vi "median filter.vi"(10 "Sample Length":i32=5, 11 "Element Input":dbl) -> (3 "Output Element":dbl)   [LabVIEW 2016]
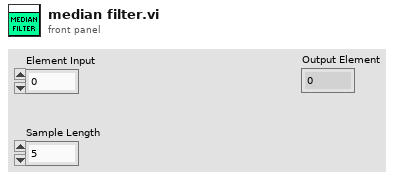
[diagram p1: front panel]
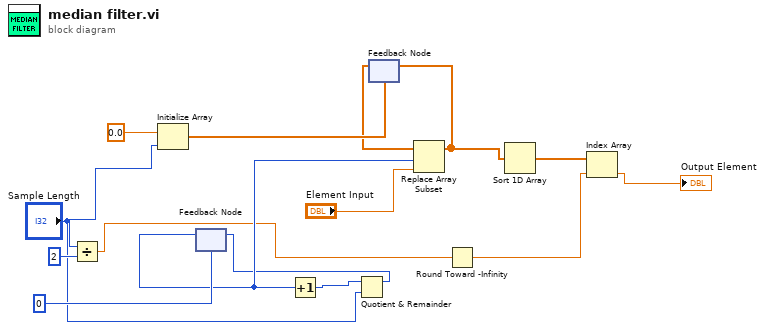
[diagram p0: block diagram]
diagram:
  n1 = Divide(x="Sample Length", y=2) -> (x/y=w5:dbl)
  n2 = Initialize Array(0.0 ("element"), "Sample Length") -> (w14:dbl[])
  n3 = feedback #1(0) -> (w9:i32)
  n4 = Increment(x=w9) -> (x+1=w11:i32)
  n5 = Quotient & Remainder(x=w11, y="Sample Length") -> (x-y*floor(x/y)=w2:i32)  [unwired: 1 out]
  n6 = feedback-in #1(w2) -> ()
  n7 = feedback #2(w14) -> (w8:dbl[])
  n8 = Replace Array Subset(array=w8, new element="Element Input", index=w9) -> (w7:dbl[])
  n9 = feedback-in #2(w7) -> ()
  n10 = Round Toward -Infinity(1:w5) -> (0:w3:dbl)
  n11 = Sort 1D Array(array=w7) -> (sorted array=w6:dbl[])
  n12 = Index Array(array=w6, index=w3) -> (element=→"Output Element":dbl)
